vi "Configure External Zero Volt Option.vi"(8 "error in (no error)":errorcluster, 10 "External Zero Volt State (False)":bool, 11 "VISA resource name":refnum<visa-resource-name>) -> (0 "error out":errorcluster, 3 "VISA resource name out":refnum<visa-resource-name>)   [LabVIEW 2017, in "HH PLI Series.lvlib"]
doc: "Enables a connection of an external Zero Volt Unit.\n\n<b>Note</b>\nConnect an external auxiliary power supply to the load terminals for using the Zero Volt ability. Please refer to the manual for that option."
uses:
  HH PLI Series.lvlib
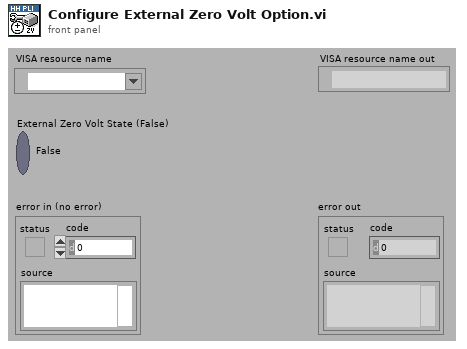
[diagram p1: front panel]
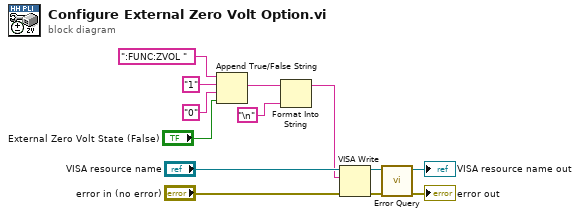
[diagram p0: block diagram]
diagram:
  n1 = Append True/False String(1:"External Zero Volt State (False)", 2:"0" ("false string"), 3:"1" ("true string"), 4:":FUNC:ZVOL " ("command")) -> (0:w2:string)
  n2 = Format Into String(initial string=w2, "\n") -> (resulting string=w1:string)  [unwired: 2 in, 1 out]
  n3 = VISA Write(VISA resource name="VISA resource name", write buffer=w1, error in (no error)="error in (no error)") -> (VISA resource name out=w6:refnum<visa-resource-name>, error out=w7:errorcluster)  [unwired: 1 out]
  n4 = call "Error Query.vi"("error in (no error)"=w7, "VISA resource name"=w6) -> ("error out"=→"error out":errorcluster, "VISA resource name out"=→"VISA resource name out":refnum<visa-resource-name>)  [unwired: 6 in, 2 out]
